vi "ex8-6.vi"   [LabVIEW 2009]
uses:
  <vilib>/NXT/Dual Mode Library/Display/NXT_Rect.ctl
  <vilib>/NXT/Dual Mode Library/Waits/Wait_Num.vi
  <vilib>/NXT/Dual Mode Library/Display/clearDisplay.vi
  <vilib>/NXT/Dual Mode Library/Display/drawRect.vi
  <vilib>/NXT/Dual Mode Library/Display/drawCircle.vi
types:
  T1 = typedef "NXT_Rect.ctl" = cluster{"Left":i16, "Bottom":i16, "Width":i16, "Height":i16}
  T2 = typedef "LVHSConnector.ctl" = cluster{"error":errorcluster, "address":string, "NXT #":i32, "Show Error":bool, "Connection":u16}
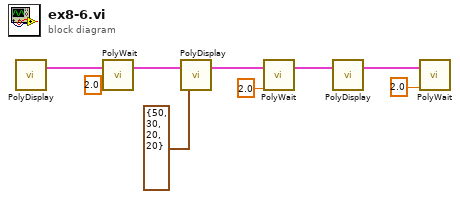
[diagram p0: block diagram]
diagram:
  n1 = call-poly <vilib>:"PolyDisplay.vi"() -> ("NXT"=w6:T2)  [unwired: 4 in]
  n2 = call-poly <vilib>:"PolyWait.vi"("Time (1 sec)"=sgl 2.0, "NXT"=w6) -> ("NXT"=w5:T2)  [unwired: 2 in]
  n3 = call-poly <vilib>:"PolyDisplay.vi"("Rect Parameters"=T1 {"Left"=50, "Bottom"=30, "Width"=20, "Height"=20}, "NXT"=w5) -> ("NXT"=w4:T2)  [unwired: 2 in]
  n4 = call-poly <vilib>:"PolyWait.vi"("Time (1 sec)"=sgl 2.0, "NXT"=w4) -> ("NXT"=w3:T2)  [unwired: 2 in]
  n5 = call-poly <vilib>:"PolyDisplay.vi"("NXT"=w3) -> ("NXT"=w2:T2)  [unwired: 3 in]
  n6 = call-poly <vilib>:"PolyWait.vi"("Time (1 sec)"=sgl 2.0, "NXT"=w2) -> ()  [unwired: 2 in, 1 out]
